vi "Launch Actor Core.vi"(7 "Host Name":string, 8 "error in (no error)":errorcluster, 9 "Actor Name":string, 10 "Message Broker":refnum<class "Message Broker Interface.lvclass">, 11 "Mediated Asynchronous Actor in":refnum<class "Mediated Asynchronous Actor.lvclass">) -> (0 "error out":errorcluster, 2 "Message Transport":refnum<class "Message Transport Interface.lvclass">)   [LabVIEW 2016, in "Stream Mediator.lvlib" / "Mediated Asynchronous Actor.lvclass"]
doc: "--\nCopyright © 2017 Composed SystemsI All rights reserved.\n\nAuthor: Jon McBee <jon.mcbee@composed.io>\n\nThis library is provided \"AS IS\" ,WITHOUT WARRANTIES OR\nCONDITIONS OF ANY KIND, either express or implied.\n\nComposed Systems -- composed.io\n\nStream 0.0.1.1\nJon McBee - Composed Systems\nCopyright (c) 2017, Composed Systems"
uses:
  <userlib>/Composed Systems/Stream/Mediator/Classes/Mediated Asynchronous Actor/Mediated Asynchronous Actor.lvclass
  <userlib>/Composed Systems/Stream/Mediator/Classes/Message Transport Interface/Message Transport Interface.lvclass
  <userlib>/Composed Systems/Stream/Mediator/Classes/Message Broker Interface/Message Broker Interface.lvclass
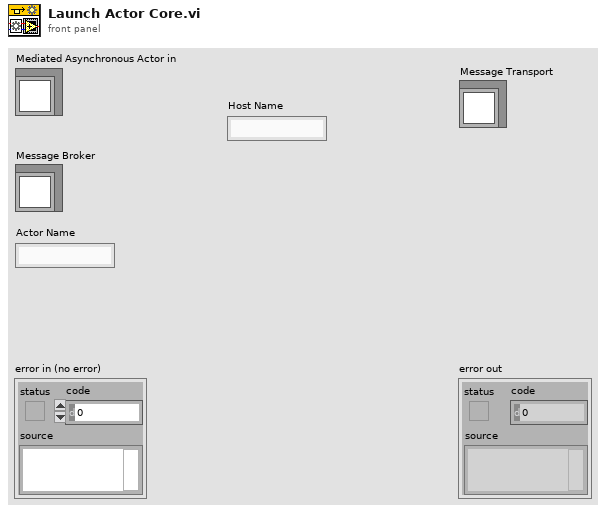
[diagram p1: front panel]
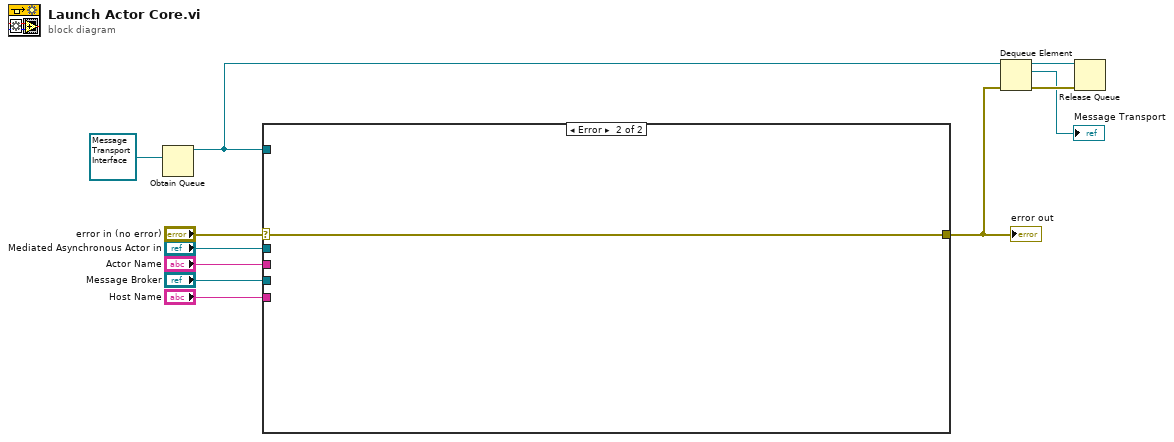
[diagram p0: block diagram]
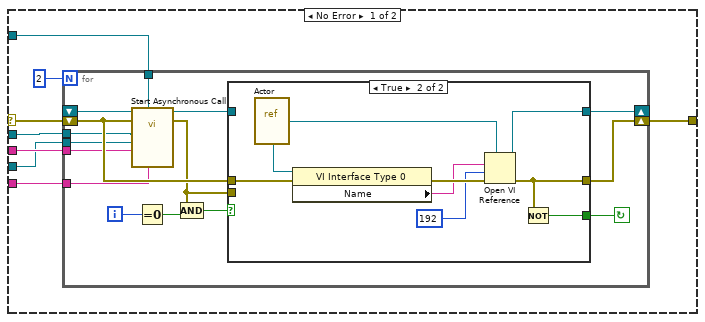
[diagram p2: hidden frame]
diagram:
  n1 = Obtain Queue(element data type=refnum<class "Message Transport Interface.lvclass"> refnum ("Message Transport Interface.lvclass")) -> (queue out=w4:refnum<queue>)  [unwired: 4 in, 2 out]
  n2 = case shown="Error" "error in (no error)" {
    selector: "error in (no error)" -> [w18 w45]
    tunnel: [w17 w45] -> w5
    tunnel: "Mediated Asynchronous Actor in" -> [w13 _]
    tunnel: w4 -> [w12 _]
    tunnel: "Host Name" -> [w16 _]
    tunnel: "Actor Name" -> [w15 _]
    tunnel: "Message Broker" -> [w14 _]
    frame No Error {
      n3 = for {
        N: 2 -> [_]
        shift-right: [w26] -> w17
        shift-left: w18 -> [w30]
        shift-right: [w27] -> _
        shift-left: _ -> [w34]
        tunnel: w16 -> [w24]
        tunnel: w15 -> [w23]
        tunnel: w14 -> [w22]
        tunnel: w13 -> [w21]
        tunnel: w12 -> [w20]
        i -> [w32]
        stop <- w25 continue-if-true
        n4 = call-by-ref "Start Asynchronous Call"(reference=w34, error in=w30, "Host Name"=w24, "Transport Queue"=w20, "Actor Name"=w23, "Message Broker Interface"=w22, "Mediated Asynchronous Actor in"=w21) -> (reference out=w33:refnum<vi>, error out=w28:errorcluster)  [unwired: 5 in, 2 out]
        n5 = Equal To 0?(x=w32) -> (x = 0?=w31:bool)
        n6 = Compound Arithmetic op=AND(w28, w31) -> (w29:bool)
        n7 = case shown="True" w29 {
          tunnel: w33 -> [w36 _]
          tunnel: w30 -> [_ w41]
          tunnel: w28 -> [w35 _]
          tunnel: [w36 w37] -> w27
          tunnel: [w35 w40] -> w26
          tunnel: [_ w39] -> w25
          frame False {
          }
          frame True {
            n8 = vi-ref <userlib>:"Actor.vi"() -> (w38:refnum<vi>)
            n9 = property class="VI Interface Type 0"(reference=w38, error in=w41) -> (error out=w44:errorcluster, "Name"=w43:string)  [unwired: 1 out]
            n10 = Open VI Reference(type specifier VI Refnum (for type only)=w38, vi path=w43, options=192, error in (no error)=w44) -> (vi reference=w37:refnum<vi>, error out=w40:errorcluster)  [unwired: 2 in]
            n11 = Not(x=w40) -> (.not. x?=w39:bool)
          }
        }
      }
    }
    frame Error {
    }
  }
  "error out" <- w5
  n12 = Dequeue Element(queue=w4, error in (no error)=w5) -> (queue out=w8:refnum<queue>, element=→"Message Transport":refnum<class "Message Transport Interface.lvclass">, error out=w7:errorcluster)  [unwired: 1 in, 1 out]
  n13 = Release Queue(queue=w8, error in (no error)=w7) -> ()  [unwired: 1 in, 3 out]
